vi "ShiftRegister.vi"() -> ()   [LabVIEW 2019]
panel:
  out "Sum Chart":dbl(graph)
  out "Final value":dbl
  out "Iterations Graph":i32[](graph)
  in  "Milliseconds\nto wait":u32
  out "Current iteration":dbl
  out "Sum":dbl
  in  "External Input":dbl
  in  "Iterations":i32
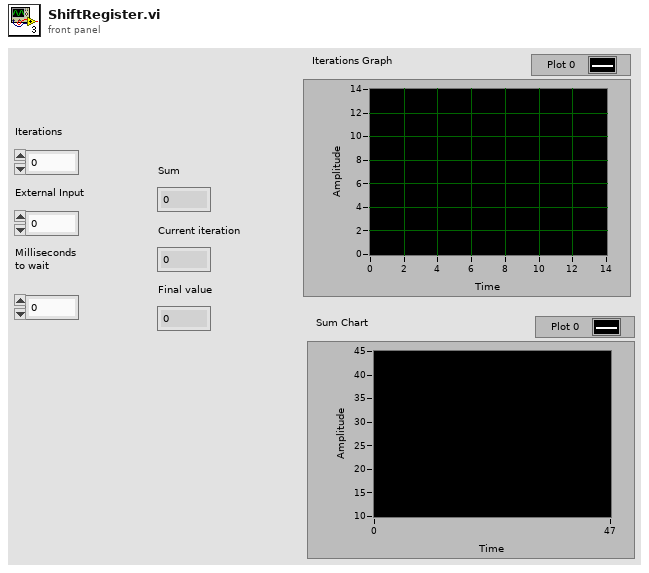
[diagram p1: front panel]
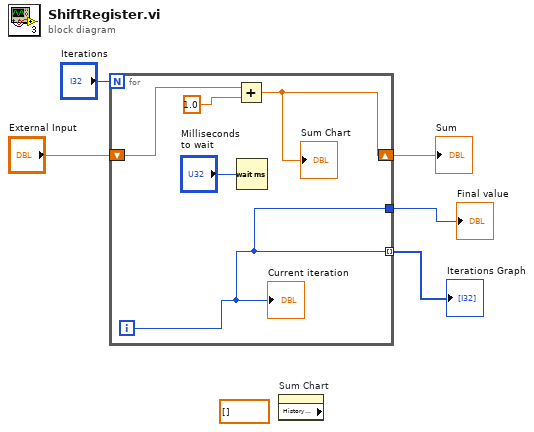
[diagram p0: block diagram]
diagram:
  (unwired) dbl[] [] ("History Data")
  n1 = for {
    N: "Iterations" -> [_]
    shift-right: [w6] -> w3
    shift-left: "External Input" -> [w8]
    tunnel: [w10] -> w1
    tunnel: [w10] -> w2 mode=indexing
    i -> [w10]
    n2 = Add(x=w8, y=1.0) -> (x+y=w6:dbl)
    "Sum Chart" <- w6
    n3 = Wait (ms)(milliseconds to wait="Milliseconds\nto wait") -> ()  [unwired: 1 out]
    "Current iteration" <- w10
  }
  "Sum" <- w3
  "Iterations Graph" <- w2
  "Final value" <- w1
  n4 = property on="Sum Chart" class="WFChart (strict)" props=["History Data"]() -> ()  [unwired: 2 in, 3 out]
